vi "process_document.vi"(0 "chunk_character_splitter in":refnum<class "chunk_character_splitter.lvclass">, 5 "documents":refnum<class "data_document.lvclass">[](array[class]), 11 "error in (no error)":errorcluster) -> (4 "chunk_character_splitter out":refnum<class "chunk_character_splitter.lvclass">, 6 "nodes":refnum<class "data_node.lvclass">[](array[class]), 15 "error out":errorcluster)   [LabVIEW 2020, in "chunk_character_splitter.lvclass"]
uses:
  chunk_character_splitter.lvclass
  data/data_document/data_document.lvclass
  data/data_node/data_node.lvclass
  chunk_character_splitter.lvclass/chunk_character_splitter.ctl
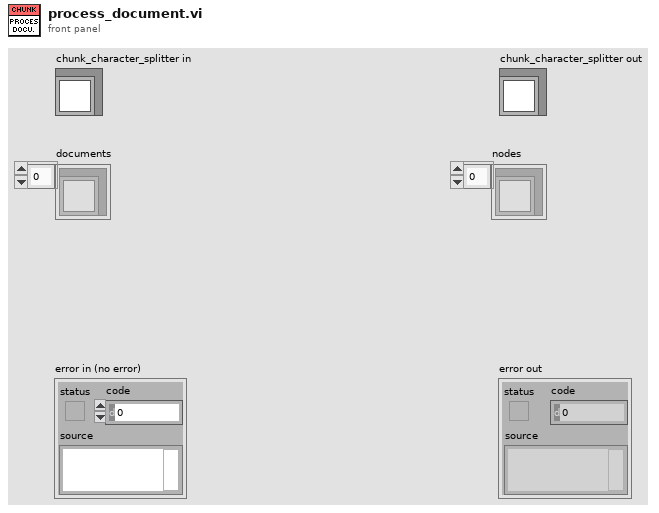
[diagram p1: front panel]
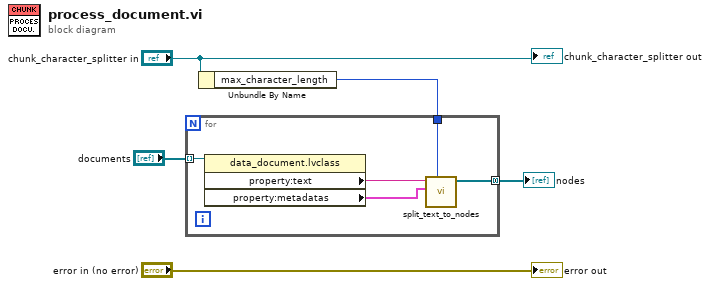
[diagram p0: block diagram]
diagram:
  n1 = Unbundle By Name("chunk_character_splitter in") -> ("max_character_length"=w3:u32)
  n2 = for {
    tunnel: "documents" -> [w10] mode=indexing
    tunnel: w3 -> [w7]
    tunnel: [w6] -> w2 mode=concatenating
    n3 = property class="data_document.lvclass"(reference=w10) -> ("property:text"=w9:string, "property:metadatas"=w8:cluster{"key":string, "value":string}[])  [unwired: 1 in, 2 out]
    n4 = call "split_text_to_nodes.vi"("max_character_length"=w7, "metadatas"=w8, "text"=w9) -> ("Nodes"=w6:refnum<class "data_node.lvclass">[])  [unwired: 8 in]
  }
  "nodes" <- w2
  "error out" <- "error in (no error)"
  "chunk_character_splitter out" <- "chunk_character_splitter in"
